vi "decodeCameras.vi"(8 "error in (no error)":errorcluster, 9 "Ignore left/rigth?":bool[](array[boolean]), 10 "unsigned byte array":u8[](array[numeric]), 11 "Vision in":refnum<class "Vision.lvclass">) -> (0 "error out":errorcluster, 1 "Field Size":T1, 2 "Detection Frame":T2 {"robots_blue"."height" format="%+4.3f"; "robots_blue"."pixel_y" format="%+4.3f"; "robots_blue"."pixel_x" format="%+4.3f"; "robots_blue"."orientation" format="%+4.3f"; "robots_blue"."y" format="%+4.3f"; "robots_blue"."confidence" format="%4.3f"; "robots_blue"."x" format="%+4.3f"; "robots_yellow"."height" format="%+4.3f"; "robots_yellow"."pixel_y" format="%+4.3f"; "robots_yellow"."pixel_x" format="%+4.3f"; "robots_yellow"."orientation" format="%+4.3f"; "robots_yellow"."y" format="%+4.3f"; "robots_yellow"."confidence" format="%4.3f"; "robots_yellow"."x" format="%+4.3f"}, 3 "Vision out":refnum<class "Vision.lvclass">, 4 "Empty Field Size?":bool, 5 "camera_id":u32, 6 "Empty Information?":bool)   [LabVIEW 2018, in "Vision.lvclass"]
uses:
  Vision.lvclass
  Old vision/Controls/SSL Detection Frame.ctl
  Old vision/Controls/SSL Detection Robot.ctl
  <vilib>/Analysis/Matrix/Datatypes/RealMatrix.ctl
  Old vision/Controls/SSL Detection Ball.ctl
  <vilib>/Analysis/Matrix/NI_Matrix.lvlib
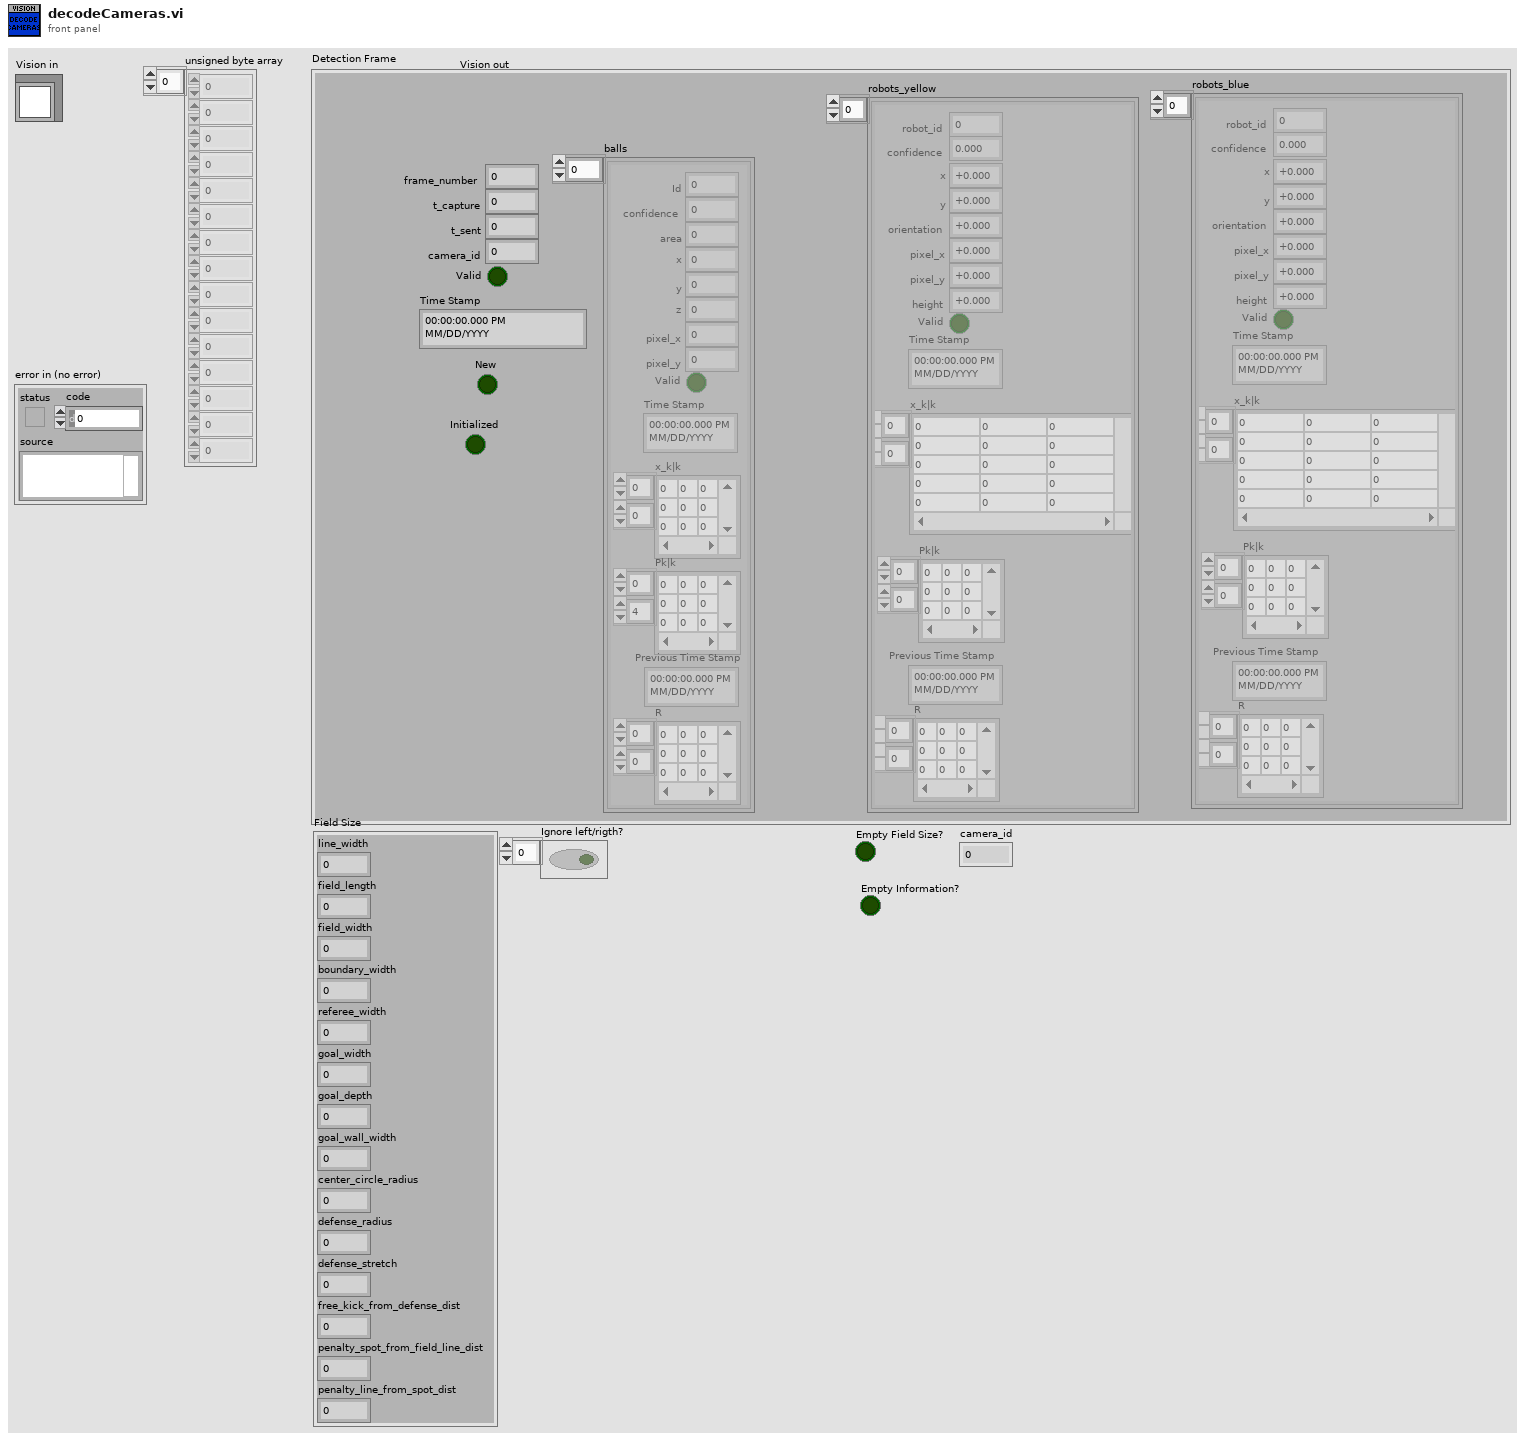
[diagram p1: front panel]
types:
  T1 = cluster{"line_width":u32, "field_length":u32, "field_width":u32, "boundary_width":u32, "referee_width":u32, "goal_width":u32, "goal_depth":u32, "goal_wall_width":u32, "center_circle_radius":u32, "defense_radius":u32, "defense_stretch":u32, "free_kick_from_defense_dist":u32, "penalty_spot_from_field_line_dist":u32, "penalty_line_from_spot_dist":u32}
  T2 = typedef "SSL Detection Frame.ctl" = cluster{"frame_number":u32, "t_capture":dbl, "t_sent":dbl, "camera_id":u32, "robots_yellow":T3[], "robots_blue":T3[], "balls":T5[], "Valid":bool, "Time Stamp":timestamp, "New":bool, "Initialized":bool}
  T3 = typedef "SSL Detection Robot.ctl" = cluster{"x":sgl, "robot_id":u32, "confidence":sgl, "y":sgl, "orientation":sgl, "pixel_x":sgl, "pixel_y":sgl, "height":sgl, "Valid":bool, "Time Stamp":timestamp, "x_k|k":T4, "Pk|k":T4, "Previous Time Stamp":timestamp, "R":T4}
  T4 = typedef "NI_Matrix.lvlib/RealMatrix.ctl" = dbl[][]
  T5 = typedef "SSL Detection Ball.ctl" = cluster{"x":sgl, "area":u32, "confidence":sgl, "y":sgl, "z":sgl, "pixel_x":sgl, "pixel_y":sgl, "Valid":bool, "Time Stamp":timestamp, "x_k|k":T4, "Pk|k":T4, "Id":u32, "Previous Time Stamp":timestamp, "R":T4}
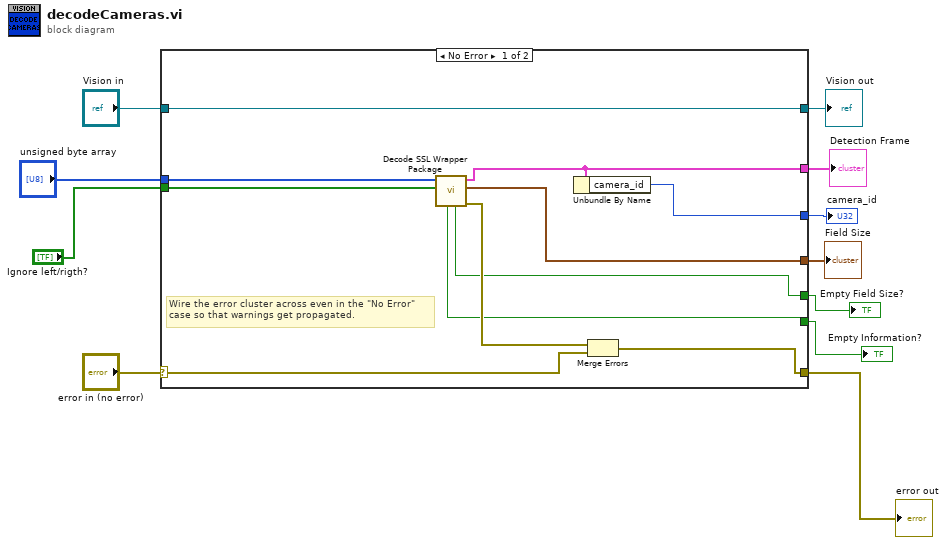
[diagram p0: block diagram]
diagram:
  n1 = case shown="No Error" "error in (no error)" {
    selector: "error in (no error)" -> [w18 w24]
    tunnel: [w17 w24] -> w10
    tunnel: [w22 w23] -> w8
    tunnel: "Vision in" -> [w22 w23]
    tunnel: "unsigned byte array" -> [w21 _]
    tunnel: [w15 _] -> w6
    tunnel: [w20 _] -> w5
    tunnel: "Ignore left/rigth?" -> [w16 _]
    tunnel: [w14 _] -> w3
    tunnel: [w13 _] -> w2
    tunnel: [w12 _] -> w1
    frame No Error {
      # "Wire the error cluster across even in the \"No Error\"\ncase so that warnings get propagated."
      n2 = call "Decode SSL Wrapper Package.vi"("Ignore left/rigth?"=w16, "unsigned byte array"=w21) -> ("error out"=w19:errorcluster, "Field Size"=w20:T1, "Detection Frame"=w15:T2, "Empty Field Size?"=w13:bool, "Empty Information?"=w12:bool)  [unwired: 4 in, 1 out]
      n3 = Unbundle By Name(w15) -> ("camera_id"=w14:u32)
      n4 = Merge Errors(w19, w18) -> (w17:errorcluster)
    }
    frame Error {
    }
  }
  "error out" <- w10
  "Vision out" <- w8
  "Detection Frame" <- w6
  "Field Size" <- w5
  "Empty Field Size?" <- w2
  "camera_id" <- w3
  "Empty Information?" <- w1
